vi "Receive - Monitor.vi"() -> ()   [LabVIEW 2020]
uses:
  src/AIM664LV.lvlib
  src/_polimorphicInstances/control/Fdx Start (Rx).vi
  src/_polimorphicInstances/session/Fdx Create Session (RX-Monitor).vi
  src/_polimorphicInstances/session/Fdx Close Session (Port).vi
  src/_polimorphicInstances/control/Fdx Stop (Rx).vi
  src/_controls/session_monitor_config.ctl
  src/_controls/monitor_becw_type.ctl
  src/_controls/monitor_fhw0_type.ctl
  src/_controls/monitor_fhw1_type.ctl
  src/_controls/monitor_entrySize_type.ctl
  src/_controls/monitor_fhInfol_type.ctl
panel:
  out "IrigTime":T1
  out "FrameHeaderInfo":T2 {"FHW0"."MacID" format="%03b"}
  out "BECW":T6
  out "Payload":u8[][](array[numeric]) format="%.0x"
  out "Synchronized":u32
  in  "EntryCount (1)":u32=1
  out "QueueStatus":T7 {"QueueStatus" items=["FDX_MON_STAT_EMPTY", "FDX_MON_STAT_ FILLED", "FDX_MON_STAT_ FULL", "FDX_MON_STAT_ OVERFLOW", "FDX_MON_STAT_ ERROR"]}
  out "current irig time":T8={"SignOut"=40, "DayOut"=1, "HourOut"=1, "MinOut"=28, "SecondOut"=39, "MilliSecOut"=539, "MicroSecOut"=300, "NanoSecOut"=0, "InfoOut"=0, "Mode"=3}
  in  "fetch period ms":u32=100
  in  "MaxFileSize MB (1)":u32=1
  in  "MonCapMode":T9 {"Strobe" items=["FDX_MON_STROBE_DIS", "FDX_MON_STROBE_STOP", "FDX_MON_STROBE_START"]; "CaptureMode" items=["FDX_MON_SINGLE ", "FDX_MON_CONTINUOUS", "FDX_MON_SELECTIVE", "FDX_MON_RECORDING", "FDX_MON_REROS", "FDX_MON_HMU"]}
  out "PortInitOut":T10={"PortConfig"=0, "PortUsed"=1, "GlobalMemFree"=0, "SharedMemFree"=0} {"PortConfig" items=["FDX_SINGLE", "FDX_REDUNDANT"]}
  in  "Port":u32=1
  in  "Board":u32
  in  "MonitorConfig":T11={"DefaultCronoMode"=2, "GlbMonBufferSizeIn"=0} {"DefaultCronoMode" items=["FDX_RX_DEFAULT_ENA_CNT", "FDX_RX_DEFAULT_MON_ENA_ALL", "FDX_RX_DEFAULT_MON_ENA_GOOD"]}
  out "error out":errorcluster
  in  "stop":bool
  out "current time":timestamp
  # "ARINC 664 Chronological Monitor"
  # "Overview: Implements a Chronological Monitor for a specific Board and Port.\n\nRequirement: One AIM ARINC-664 board with installed AIM ARINC 664 BSP.\nRestrictions: None.\nInstruction:\n1. Select the Board ID (0 if you have only one board in your system).\n2. Run the VI.\n3. See the result in Current IRIG Time"
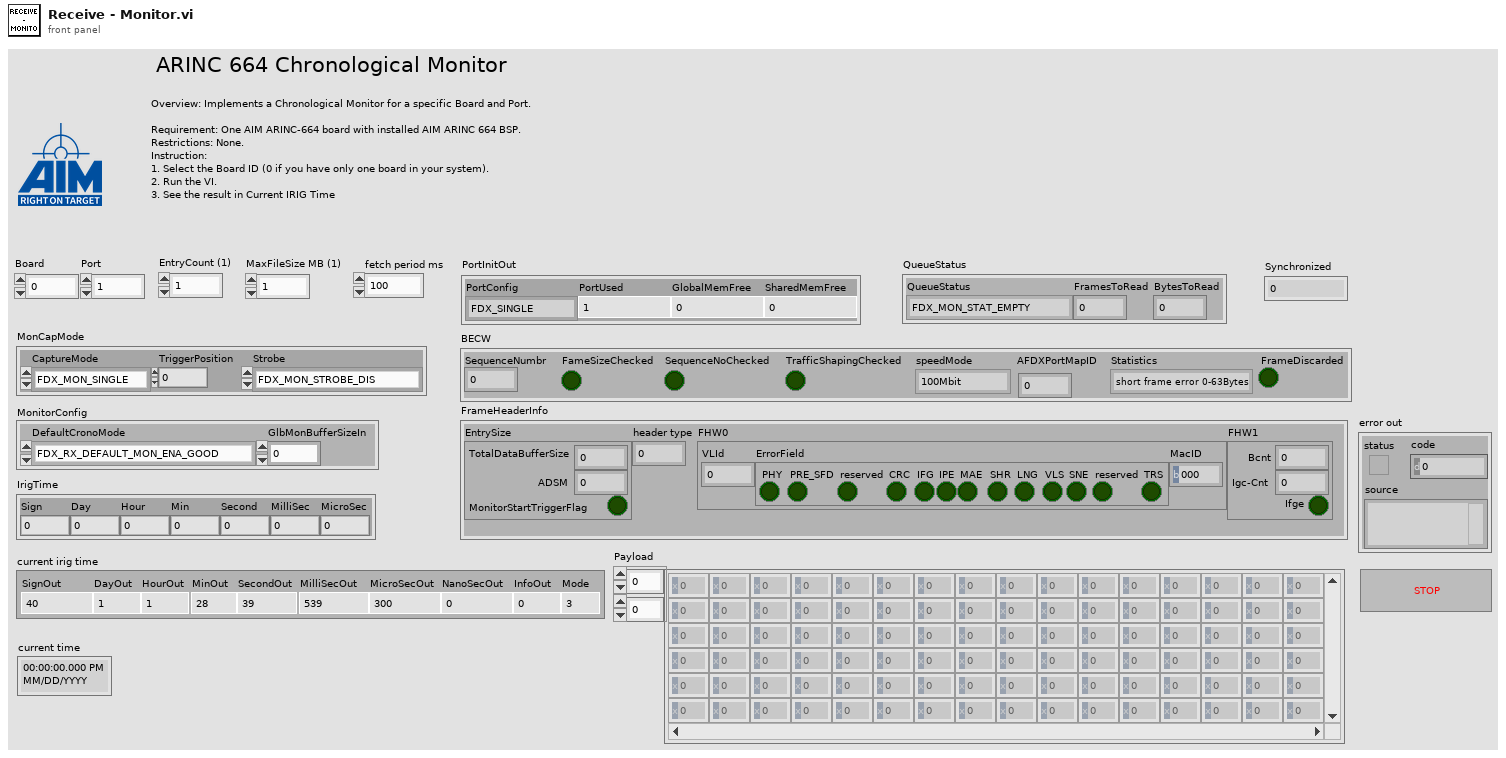
[diagram p1: front panel]
types:
  T1 = cluster{"Sign":i32, "Hour":u32, "Min":u32, "Second":u32, "Day":u32, "MilliSec":u32, "MicroSec":u32}
  T2 = typedef "AIM664LV.lvlib/monitor_fhInfol_type.ctl" = cluster{"EntrySize":T3, "header type":u32, "FHW0":T4, "FHW1":T5}
  T3 = typedef "AIM664LV.lvlib/monitor_entrySize_type.ctl" = cluster{"TotalDataBufferSize":u16, "ADSM":u16, "MonitorStartTriggerFlag":bool}
  T4 = typedef "AIM664LV.lvlib/monitor_fhw0_type.ctl" = cluster{"VLId":u16, "ErrorField":cluster{"PHY":bool, "PRE_SFD":bool, "reserved":bool, "CRC":bool, "IFG":bool, "IPE":bool, "MAE":bool, "SHR":bool, "LNG":bool, "VLS":bool, "SNE":bool, "reserved":bool, "TRS":bool}, "MacID":u8}
  T5 = typedef "AIM664LV.lvlib/monitor_fhw1_type.ctl" = cluster{"Bcnt":u16, "Igc-Cnt":u16, "Ifge":bool}
  T6 = typedef "AIM664LV.lvlib/monitor_becw_type.ctl" = cluster{"SequenceNumbr":u8, "FameSizeChecked":bool, "SequenceNoChecked":bool, "TrafficShapingChecked":bool, "speedMode":enum16{"100Mbit", "10Mbit", "1Gbit"}, "AFDXPortMapID":u8, "Statistics":enum16{"short frame error 0-63Bytes", "64-127 Bytes", "128-255 Bytes", "256-511 Bytes", "512-1023 Bytes", "1024-1518 Bytes", ">1518 Bytes"}, "FrameDiscarded":bool}
  T7 = cluster{"QueueStatus":u32, "FramesToRead":u32, "BytesToRead":u32}
  T8 = cluster{"SignOut":i32, "DayOut":u32, "HourOut":u32, "MinOut":u32, "SecondOut":u32, "MilliSecOut":u32, "MicroSecOut":u32, "NanoSecOut":u32, "InfoOut":u32, "Mode":u32}
  T9 = cluster{"CaptureMode":u32, "TriggerPosition":u32, "Strobe":u32}
  T10 = cluster{"PortConfig":u32, "PortUsed":u32, "GlobalMemFree":u32, "SharedMemFree":u32}
  T11 = typedef "AIM664LV.lvlib/session_monitor_config.ctl" = cluster{"DefaultCronoMode":u32, "GlbMonBufferSizeIn":u32}
  T12 = cluster{"EntryRead":u32, "BytesRead":u32, "Synchronized":u32, "ReadBuffer":u8[]}
  T13 = typedef "AIM664LV.lvlib/IrigTime.ctl" = cluster{"Sign":i32, "Day":u32, "Hour":u32, "Min":u32, "Second":u32, "MilliSec":u32, "MicroSec":u32}
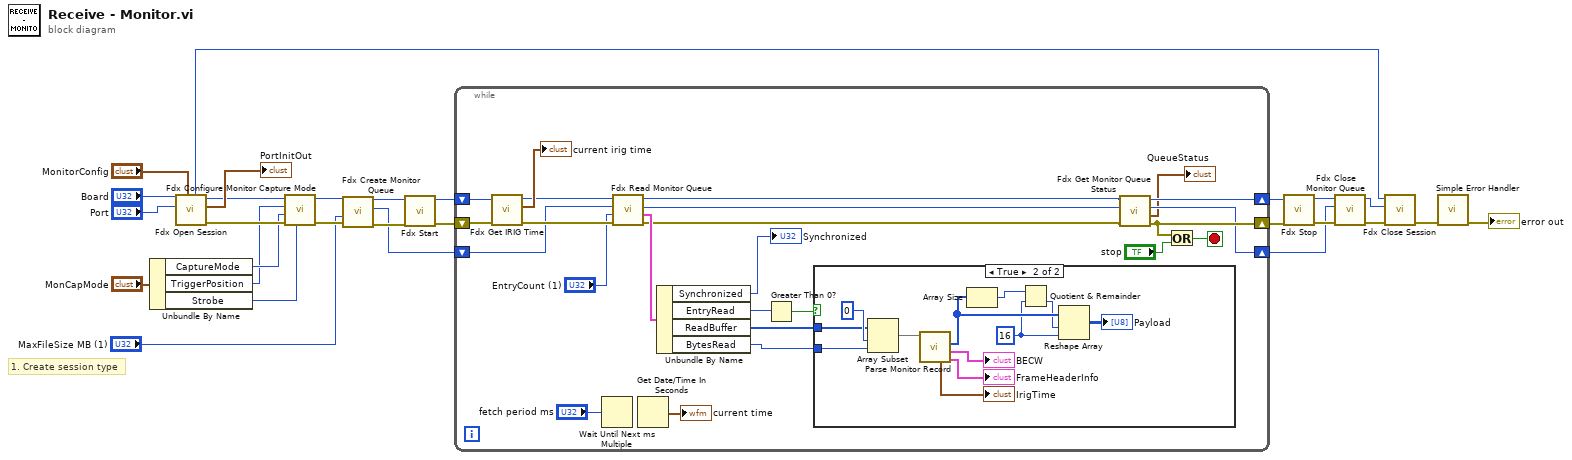
[diagram p0: block diagram]
diagram:
  # "1. Create session type"
  n1 = Unbundle By Name("MonCapMode") -> ("CaptureMode"=w9:u32, "TriggerPosition"=w8:u32, "Strobe"=w7:u32)
  n2 = call-poly "Fdx Open Session.vi"("MonitorConfig"="MonitorConfig", "port"="Port", "board"="Board") -> ("error out"=w20:errorcluster, "PortInitOut"=→"PortInitOut":T10, "InstrumentHandle_port out"=w21:u32, "InstrumentHandle_board out"=w12:u32)  [unwired: 3 in, 2 out]
  n3 = call "Fdx Configure Monitor Capture Mode.vi"("Strobe"=w7, "error in (no error)"=w20, "CaptureMode"=w9, "TriggerPosition"=w8, "InstrumentHandle_port in"=w21) -> ("error out"=w19:errorcluster, "InstrumentHandle_port out"=w18:u32)  [unwired: 5 in]
  n4 = call "Fdx Create Monitor Queue.vi"("error in (no error)"=w19, "MaxFileSize MB (1)"="MaxFileSize MB (1)", "InstrumentHandle_port in"=w18) -> ("error out"=w16:errorcluster, "QueueIdOut"=w15:u32, "InstrumentHandle_port out"=w17:u32)  [unwired: 5 in, 1 out]
  n5 = call-poly "Fdx Start.vi"("error in (no error)"=w16, "InstrumentHandle_port in"=w17) -> ("error out"=w26:errorcluster, "InstrumentHandle_port out"=w28:u32)  [unwired: 8 in]
  n6 = while {
    shift-right: [w32] -> w27
    shift-left: w28 -> [w49]
    shift-right: [w36] -> w25
    shift-left: w26 -> [w48]
    shift-right: [w31] -> w4
    shift-left: w15 -> [w33]
    stop <- w50 stop-if-true
    n7 = call "Fdx Get IRIG Time.vi"("error in (no error)"=w48, "InstrumentHandle_board in"=w49) -> ("error out"=w45:errorcluster, "Curent Irig Time"=→"current irig time":T8, "InstrumentHandle_board out"=w34:u32)  [unwired: 7 in]
    n8 = Wait Until Next ms Multiple(millisecond multiple="fetch period ms") -> ()  [unwired: 1 out]
    n9 = call "Fdx Read Monitor Queue.vi"("error in (no error)"=w45, "EntryCount (1)"="EntryCount (1)", "QueueId in"=w33, "InstrumentHandle_port in"=w34) -> ("error out"=w37:errorcluster, "QueueReadOut"=w43:T12, "QueueId out"=w29:u32, "InstrumentHandle_port out"=w38:u32)  [unwired: 4 in]
    n10 = Get Date/Time In Seconds() -> (seconds since 1Jan1904=→"current time":timestamp)
    n11 = Unbundle By Name(w43) -> ("Synchronized"=→"Synchronized":u32, "EntryRead"=w42:u32, "ReadBuffer"=w40:u8[], "BytesRead"=w39:u32)
    n12 = Greater Than 0?(x=w42) -> (x > 0?=w44:bool)
    n13 = case shown="True" w44 {
      tunnel: w40 -> [_ w60]
      tunnel: w39 -> [_ w59]
      frame False {
      }
      frame True {
        w54 = 16 ("dimension size")
        n14 = Array Subset(array=w60, index=0, length=w59) -> (w58:u8[])
        n15 = call "Parse Monitor Record.vi"("Record In"=w58) -> ("FrameHeaderInfo"=→"FrameHeaderInfo":T2, "BECW"=→"BECW":T6, "Payload"=w57:u8[], "IrigTime"=→"IrigTime":T13)  [unwired: 5 in, 2 out]
        n16 = Array Size(array=w57) -> (size(s)=w55:i32)
        n17 = Quotient & Remainder(x=w55, y=w54) -> (floor(x/y)=w53:i32)  [unwired: 1 out]
        n18 = Reshape Array(w57, w53, w54) -> (→"Payload":u8[][])
      }
    }
    n19 = call "Fdx Get Monitor Queue Status.vi"("error in (no error)"=w37, "QueueId in"=w29, "InstrumentHandle_port in"=w38) -> ("error out"=w36:errorcluster, "QueueStatus"=→"QueueStatus":T7, "QueueId out"=w31:u32, "InstrumentHandle_port out"=w32:u32)  [unwired: 5 in]
    n20 = Or(x=w36, y="stop") -> (x .or. y?=w50:bool)
  }
  n21 = call-poly "Fdx Stop.vi"("error in (no error)"=w25, "InstrumentHandle_port in"=w27) -> ("error out"=w14:errorcluster, "InstrumentHandle_port out"=w6:u32)  [unwired: 8 in]
  n22 = call "Fdx Close Monitor Queue.vi"("error in (no error)"=w14, "QueueId"=w4, "InstrumentHandle_port in"=w6) -> ("error out"=w13:errorcluster, "InstrumentHandle_port out"=w5:u32)  [unwired: 7 in]
  n23 = call-poly "Fdx Close Session.vi"("error in (no error)"=w13, "InstrumentHandle_port in"=w5, "InstrumentHandle_board in"=w12) -> ("error out"=w2:errorcluster)  [unwired: 8 in]
  n24 = call <vilib>:"Simple Error Handler.vi"("error in (no error)"=w2) -> ("error out"=→"error out":errorcluster)  [unwired: 4 in, 4 out]
